vi "Cascade Lowpass and Highpass to Bandpass Filter.vi"() -> ()   [LabVIEW 2023]
doc: "Demonstrates how to use the DFD Cascade Filters VI to cascade two filters into one filter. The two filters are lowpass and highpass filters, respectively. The resulting filter is a bandpass filter. The transfer function of the bandpass filter is the transfer function convolution of the lowpass and highpass filters you cascade. \n\nComplete the following steps to use this VI.\n1) Run the VI.\n2) Observe the Magnitude Response graph to verify that the <B>Cascaded Bandpass</B> plot is the sum of the <B>Lowpass</B> plot and the <B>Highpass</B> plot in dB."
uses:
  <vilib>/addons/Digital Filter Design/_Objects.llb/DFD Filter Frequence Specification (Design).ctl
  <vilib>/addons/Digital Filter Design/Analysis.llb/DFD Plot Freq Response (Linear-Spaced).vi
  <vilib>/addons/Digital Filter Design/NI_DigFilterLicensed.lvlib
panel:
  in  "Sampling Frequency [Hz]":dbl=1.0 format="%.2f"
  in  "fstop_hp":dbl=0.1 caption="Stopband Frequency [Hz]"
  in  "fpass_hp":dbl=0.2 caption="Passband Frequency [Hz]"
  in  "fstop_lp":dbl=0.45 caption="Stopband Frequency [Hz]"
  in  "fpass_lp":dbl=0.4 caption="Passband Frequency [Hz]"
  out "Error Message":string
  out "Magnitude Response":cluster{"f0":dbl, "df":dbl, "magnitude":dbl[]}[](graph)
  # "Select Help>>Show Context Help and move the cursor over the VI icon for more information."
  # "Lowpass Specifications"
  # "Highpass Specifications"
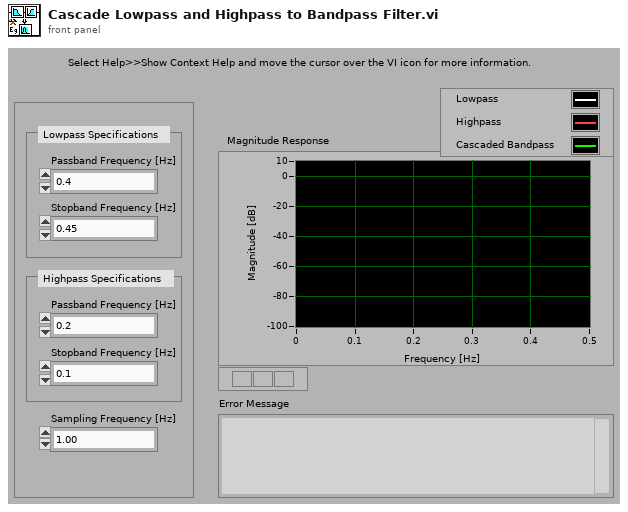
[diagram p1: front panel]
types:
  T1 = typedef "NI_DigFilterLicensed.lvlib/DFD Filter Frequence Specification (Design).ctl" = cluster{"fpass 1":dbl, "fstop 1":dbl, "fpass 2 ":dbl, "fstop 2":dbl}
  T2 = enum16{"Lowpass", "Highpass", "Bandpass", "Bandstop"}
  T3 = typedef "NI_DigFilterLicensed.lvlib/DFD Filter Obj.ctl" = cluster{"mSRate_Fs":dbl, "mSRate_Version":string, "mSRate_Comments":string, "mSRate_OrgCoef":T4, "mSRate_CurCoef":T4, "mSRate_Quantized?":bool, "mSRate_QCoef":T4, "mSRate_QSettings":T6[], "mSRate_Order":i32, "mSRate_Scaling":cluster{"mSRate_ScaleByPowerOf2?":bool, "mSRate_ScaleType":T8}}
  T4 = typedef "NI_DigFilterLicensed.lvlib/DFD Filter Coef.ctl" = cluster{"type":T5, "gain":dbl, "coef a (k)":dbl[], "coef b (v)":dbl[]}
  T5 = typedef "NI_DigFilterLicensed.lvlib/DFD Filter Structure Type Selector.ctl" = enum16{"Undefined", "FIR Direct Form", "FIR Direct Form Transposed", "FIR Symmetric", "FIR Antisymmetric", "IIR Direct Form I", "IIR Direct Form I Transposed", "IIR Direct Form II", "IIR Direct Form II Transposed", "IIR Cascaded Second Order Sections Form I", "IIR Cascaded Second Order Sections Form I Transposed", "IIR Cascaded Second Order Sections Form II", "IIR Cascaded Second Order Sections Form II Transposed", "Lattice Allpass (basic sections)", "Lattice Allpass (one multiplier sections)", "Lattice Allpass (normalized sections)", "Lattice AR (basic sections)", "Lattice AR (one multiplier sections)", "Lattice AR (normalized sections)", "Lattice MA (minimum phase)", "Lattice MA (maximum phase)", "Lattice ARMA (basic sections)", "Lattice ARMA (one multiplier sections)", "Lattice ARMA (normalized sections)"}
  T6 = typedef "NI_DigFilterLicensed.lvlib/dfd_Internal Quantization Settings.ctl" = cluster{"source":T7, "wl":i16, "iwl":i16, "overflow mode":enum16{"Saturation", "Wrap"}, "rounding mode":enum16{"Nearest", "Truncation"}, "signed?":bool}
  T7 = typedef "NI_DigFilterLicensed.lvlib/dfd_Internal Quantization Srcs.ctl" = u16
  T8 = typedef "NI_DigFilterLicensed.lvlib/DFD Coef Norm Type.ctl" = enum16{"No Norm", "Time Domain 1-Norm", "Time Domain 2-Norm", "Time Domain Inf-Norm"}
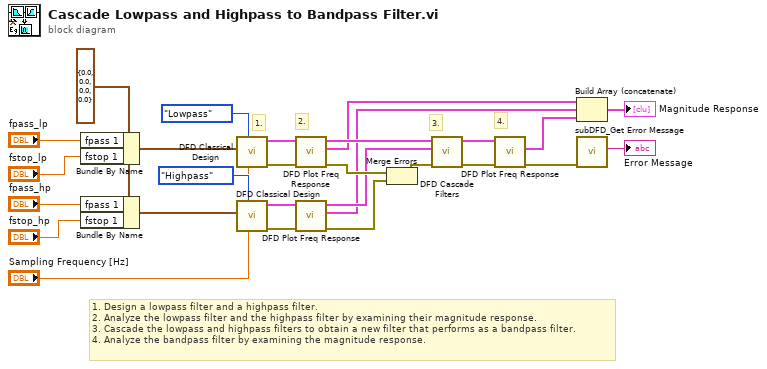
[diagram p0: block diagram]
diagram:
  w6 = T1 {"fpass 1"=0.0, "fstop 1"=0.0, "fpass 2 "=0.0, "fstop 2"=0.0} ("Frequency Specifications [Hz]")
  # "4."
  # "3."
  # "2."
  # "1."
  # "1. Design a lowpass filter and a highpass filter.\n2. Analyze the lowpass filter and the highpass filter by examining their magnitude response.\n3. Cascade the lowpass and highpass filters to obtain a new filter that performs as a bandpass filter. \n4. Analyze the bandpass filter by examining the magnitude response."
  n1 = Bundle By Name(cluster=w6, "fpass 1"="fpass_lp", "fstop 1"="fstop_lp") -> (w8:T1)
  n2 = Bundle By Name(cluster=w6, "fpass 1"="fpass_hp", "fstop 1"="fstop_hp") -> (w7:T1)
  n3 = call <vilib>:"DFD Classical Design.vi"("fs [Hz]"="Sampling Frequency [Hz]", "filter type"=T2."Lowpass", "freq specs [Hz]"=w8) -> ("error out"=w22:errorcluster, "filter out"=w23:T3)  [unwired: 3 in, 4 out]
  n4 = call <vilib>:"DFD Classical Design.vi"("fs [Hz]"="Sampling Frequency [Hz]", "filter type"=T2."Highpass", "freq specs [Hz]"=w7) -> ("error out"=w20:errorcluster, "filter out"=w21:T3)  [unwired: 3 in, 4 out]
  n5 = call-poly <vilib>:"DFD Plot Freq Response.vi"("error in (no error)"=w22, "filter in"=w23) -> ("magnitude response"=w13:cluster{"f0":dbl, "df":dbl, "values":dbl[]}[])  [unwired: 6 in, 3 out]
  n6 = call-poly <vilib>:"DFD Plot Freq Response.vi"("error in (no error)"=w20, "filter in"=w21) -> ("error out"=w18:errorcluster, "magnitude response"=w12:cluster{"f0":dbl, "df":dbl, "values":dbl[]}[], "filter out"=w19:T3)  [unwired: 6 in, 1 out]
  n7 = Merge Errors(w22, w18) -> (w17:errorcluster)
  n8 = call <vilib>:"DFD Cascade Filters.vi"("error in (no error)"=w17, "filter in 2"=w19, "filter in 1"=w23) -> ("error out"=w16:errorcluster, "filter out"=w15:T3)  [unwired: 1 in, 6 out]
  n9 = call-poly <vilib>:"DFD Plot Freq Response.vi"("error in (no error)"=w16, "filter in"=w15) -> ("error out"=w9:errorcluster, "magnitude response"=w14:cluster{"f0":dbl, "df":dbl, "values":dbl[]}[])  [unwired: 6 in, 2 out]
  n10 = Build Array (concatenate)(w13, w12, w14) -> (→"Magnitude Response":cluster{"f0":dbl, "df":dbl, "values":dbl[]}[])
  n11 = call <vilib>:"subDFD_Get Error Message.vi"("error in (no error)"=w9) -> ("Error Message"=→"Error Message":string)  [unwired: 10 out]
